vi "Pointer.In-Place Read (1D I16).vi"(8 "error in (no error)":errorcluster, 10 "allocated array in":i16[](array[numeric]), 11 "pointer in":u64) -> (0 "error out":errorcluster, 2 "array out":i16[](array[numeric]), 3 "pointer out":u64)   [LabVIEW 2016, in "VeriStand Data.lvlib"]
doc: "Reads a number of values, specified by the size of the provided <B>array</B>, from the provided <B>pointer</B>."
uses:
  VeriStand Data.lvlib
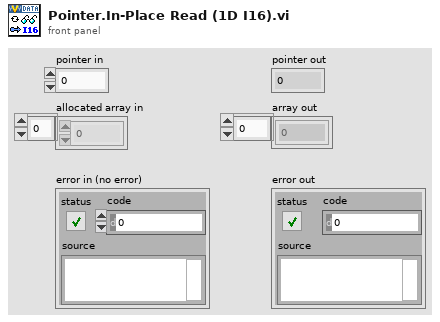
[diagram p1: front panel]
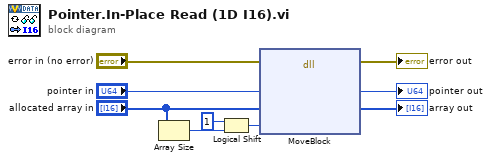
[diagram p0: block diagram]
diagram:
  n1 = Array Size(array="allocated array in") -> (size(s)=w1:i32)
  n2 = Logical Shift(y=i16 1, x=w1) -> (x << y=w3:i32)
  n3 = dll-call lib="LabVIEW" fn="MoveBlock"(error in="error in (no error)", "ps"="pointer in", "pd"="allocated array in", "size"=w3) -> (error out=→"error out":errorcluster, "ps"=→"pointer out":u64, "pd"=→"array out":i16[])  [unwired: 4 in, 1 out]
